vi "Clear Arbitrary Memory [SEQ].vi"(8 "error in (no error)":errorcluster, 11 "CS++Fgen in":refnum<class "CS++Fgen.lvclass">) -> (0 "error out":errorcluster, 3 "CS++Fgen out":refnum<class "CS++Fgen.lvclass">)   [LabVIEW 2013, in "CS++Fgen.lvlib" / "CS++Fgen.lvclass"]
doc: "This VI removes all previously created arbitrary waveforms and sequences from the function generator's memory. It also invalidates all waveform and sequence handles.\n\nNotes:\n\n(1) This VI is part of the IviFgenArbSeq [SEQ] extension group."
uses:
  CS++Fgen.lvclass
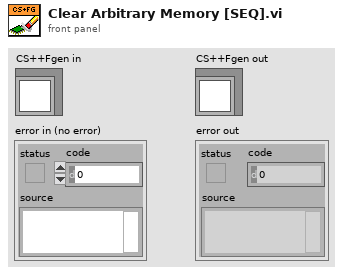
[diagram p1: front panel]
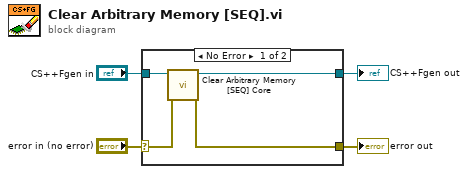
[diagram p0: block diagram]
diagram:
  n1 = case shown="No Error" "error in (no error)" {
    selector: "error in (no error)" -> [w6 w10]
    tunnel: [w5 w10] -> w3
    tunnel: [w7 w9] -> w1
    tunnel: "CS++Fgen in" -> [w8 w9]
    frame No Error {
      n2 = call-dynamic "Clear Arbitrary Memory [SEQ] Core.vi"("error in (no error)"=w6, "CS++Fgen in"=w8) -> ("error out"=w5:errorcluster, "CS++Fgen out"=w7:refnum<class "CS++Fgen.lvclass">)  [unwired: 8 in]
    }
    frame Error {
    }
  }
  "error out" <- w3
  "CS++Fgen out" <- w1
